vi "getOutputState.vi"(8 "error in (no error)":errorcluster, 10 "Channel Nr (1)":string="1", 11 "VISA resource name":refnum<visa-resource-name>) -> (0 "error out":errorcluster, 2 "Output State":bool, 3 "VISA resource name out":refnum<visa-resource-name>)   [LabVIEW 2023, in "Tti-Pl303Qmd.lvlib"]
doc: "Get output state of channel"
uses:
  Tti-Pl303Qmd.lvlib
  <vilib>/Utility/error.llb/Error Cluster From Error Code.vi
  <vilib>/ErrorRing/Error Ring.xnode
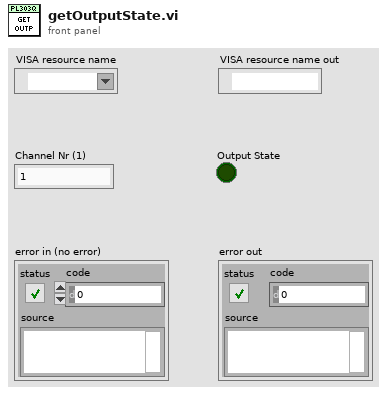
[diagram p1: front panel]
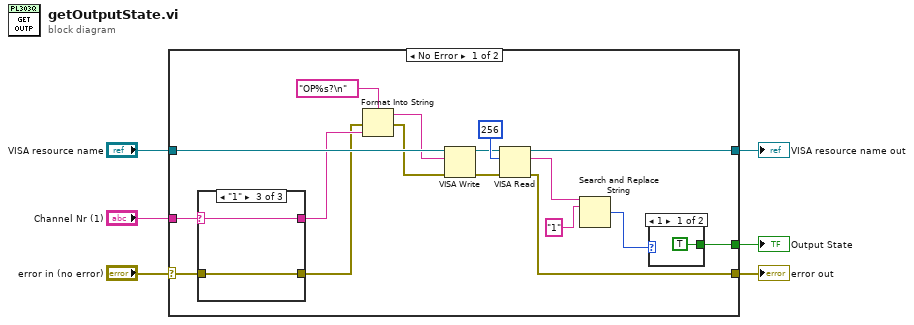
[diagram p0: block diagram]
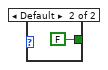
[diagram p2: hidden frame]
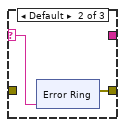
[diagram p4: hidden frame]
diagram:
  n1 = case shown="No Error" "error in (no error)" {
    selector: "error in (no error)" -> [w21 w40]
    tunnel: "VISA resource name" -> [w23 w39]
    tunnel: [w11 w40] -> w2
    tunnel: "Channel Nr (1)" -> [w22 _]
    tunnel: [w13 w39] -> w3
    tunnel: [w10 _] -> w1
    frame No Error {
      n2 = case shown="\"1\"" w22 {
        selector: w22 -> [w27 w28 w37]
        tunnel: w21 -> [w26 _ w38]
        tunnel: [w26 w29 w38] -> w18
        tunnel: [w27 _ w37] -> w19
        frame "2" {
        }
        frame Default {
          n3 = xnode "Error Ring"("parameter 0"=w28) -> ("error out"=w29:errorcluster)
        }
        frame "1" {
        }
      }
      n4 = Format Into String(format string="OP%s?\n" ("write buffer"), error in=w18, w19) -> (resulting string=w16:string, error out=w17:errorcluster)  [unwired: 1 in]
      n5 = VISA Write(VISA resource name=w23, write buffer=w16, error in (no error)=w17) -> (VISA resource name out=w12:refnum<visa-resource-name>, error out=w15:errorcluster)  [unwired: 1 out]
      n6 = VISA Read(VISA resource name=w12, byte count=u32 256, error in (no error)=w15) -> (VISA resource name out=w13:refnum<visa-resource-name>, read buffer=w9:string, error out=w11:errorcluster)  [unwired: 1 out]
      n7 = Search and Replace String(input string=w9, search string="1") -> (number of replacements=w7:i32)  [unwired: 6 in, 3 out]
      n8 = case shown="1" w7 {
        tunnel: [TRUE FALSE] -> w10
        frame 1 {
        }
        frame Default {
        }
      }
    }
    frame Error {
    }
  }
  "error out" <- w2
  "VISA resource name out" <- w3
  "Output State" <- w1
